vi "Result Response.vi"(8 "error in (no error)":errorcluster, 10 "Acquired Result.lvclass":refnum<class "Acquired Result.lvclass">, 11 "Monitor Controller in":refnum<class "Monitor Controller.lvclass">) -> (0 "error out":errorcluster, 3 "Monitor Controller out":refnum<class "Monitor Controller.lvclass">)   [LabVIEW 2016, in "Monitor Controller.lvclass"]
uses:
  Monitor Controller.lvclass
  D:/github/Measure_core/Da Base/Da Base.lvclass
  D:/Program Files/National Instruments/LabVIEW 2016/vi.lib/ActorFramework/Actor/Actor.lvclass
  Results/Acquired Result/Acquired Result.lvclass
  Monitor Controller.lvclass/Monitor Controller.ctl
  Da Base/Da Base.lvclass/Da Base.ctl
  <vilib>/ActorFramework/Actor/Actor.lvclass/Actor.ctl
  Process Controller Messages/Update Plots Msg/Update Plots Msg.lvclass/Update Plots Msg.ctl
  <vilib>/ActorFramework/Message Enqueuer/Message Enqueuer.lvclass/Message Enqueuer.ctl
  da Base/Read tdms stream.vi
  <vilib>/ActorFramework/Message Enqueuer/Enqueue.vi
  Process Controller Messages/Update Plots Msg/Update Plots Msg.lvclass
  D:/Program Files/National Instruments/LabVIEW 2016/vi.lib/ActorFramework/Message/Message.lvclass
  Read Monitor controller configuration.vi
  <vilib>/ActorFramework/Message Priority Queue/Priority Enqueue.vi
  Process Controller/Process Controller.lvclass
  <vilib>/ActorFramework/Actor/Actor.lvclass
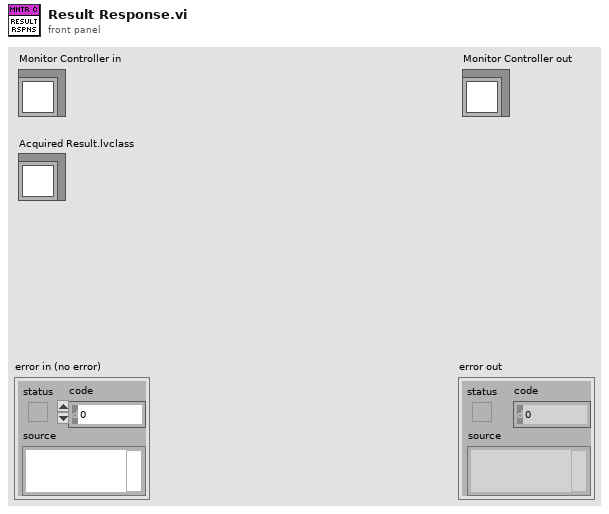
[diagram p1: front panel]
types:
  T1 = typedef "Monitor Controller Configuration.ctl" = cluster{"Period":dbl, "Repeat times":i32, "Open plot":bool, "File defragment period":dbl}
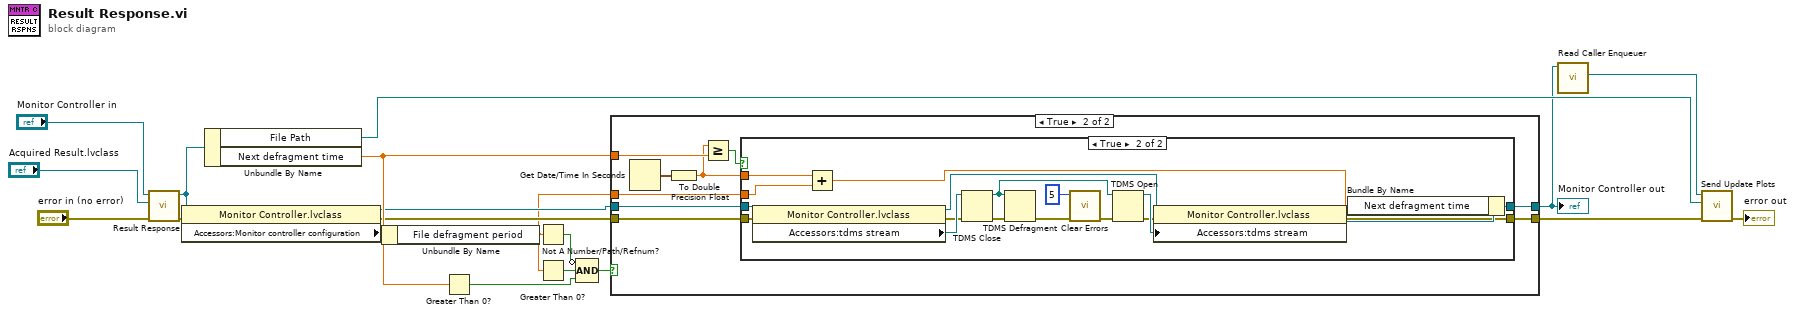
[diagram p0: block diagram]
diagram:
  n1 = call-parent "Result Response.vi"("error in (no error)"="error in (no error)", "Acquired Result"="Acquired Result.lvclass", "Measure Controller in"="Monitor Controller in") -> ("error out"=w2:errorcluster, "Measure Controller out"=w14:refnum<class "Monitor Controller.lvclass">)  [unwired: 7 in]
  n2 = property class="Monitor Controller.lvclass"(reference=w14, error in=w2) -> (reference out=w7:refnum<class "Monitor Controller.lvclass">, error out=w6:errorcluster, "Accessors:Monitor controller configuration"=w13:T1)
  n3 = Unbundle By Name(w14) -> ("File Path"=w15:path, "Next defragment time"=w8:dbl)
  n4 = Unbundle By Name(w13) -> ("File defragment period"=w5:dbl)
  n5 = Greater Than 0?(x=w8) -> (x > 0?=w9:bool)
  n6 = Not A Number/Path/Refnum?(number/path/refnum=w5) -> (NaN/Path/Refnum?=w11:bool)
  n7 = Greater Than 0?(x=w5) -> (x > 0?=w12:bool)
  n8 = Compound Arithmetic op=AND(invert w11, w12, w9) -> (w10:bool)
  n9 = case shown="True" w10 {
    tunnel: w8 -> [_ w29]
    tunnel: w7 -> [w21 w27]
    tunnel: w6 -> [w20 w26]
    tunnel: w5 -> [_ w24]
    tunnel: [w21 w23] -> w1
    tunnel: [w20 w22] -> w4
    frame False {
    }
    frame True {
      n10 = Get Date/Time In Seconds() -> (seconds since 1Jan1904=w30:timestamp)
      n11 = To Double Precision Float(number=w30) -> (double precision float=w25:dbl)
      n12 = Greater Or Equal?(x=w25, y=w29) -> (x >= y?=w28:bool)
      n13 = case shown="True" w28 {
        tunnel: w27 -> [w32 w50]
        tunnel: w26 -> [w31 w49]
        tunnel: w25 -> [_ w40]
        tunnel: w24 -> [_ w39]
        tunnel: [w32 w36] -> w23
        tunnel: [w31 w35] -> w22
        frame False {
        }
        frame True {
          n14 = property class="Monitor Controller.lvclass"(reference=w50, error in=w49) -> (reference out=w43:refnum<class "Monitor Controller.lvclass">, error out=w47:errorcluster, "Accessors:tdms stream"=w48:refnum<k34>)
          n15 = Add(x=w40, y=w39) -> (x+y=w37:dbl)
          n16 = TDMS Close(8:w47, 11:w48) -> (0:w46:errorcluster, 3:w44:path)
          n17 = TDMS Defragment(4:w46, 7:w44) -> (0:w45:errorcluster)
          n18 = call <vilib>:"Clear Errors.vi"("error in (no error)"=w45, "specific error code to clear (0: all)"=5) -> ("error out"=w34:errorcluster)  [unwired: 4 in, 1 out]
          n19 = TDMS Open(8:w34, 11:w44) -> (0:w41:errorcluster, 3:w42:refnum<k34>)  [unwired: 5 in]
          n20 = property class="Monitor Controller.lvclass"(reference=w43, error in=w41, "Accessors:tdms stream"=w42) -> (reference out=w38:refnum<class "Monitor Controller.lvclass">, error out=w35:errorcluster)
          n21 = Bundle By Name(cluster=w38, "Next defragment time"=w37) -> (w36:refnum<class "Monitor Controller.lvclass">)
        }
      }
    }
  }
  "Monitor Controller out" <- w1
  n22 = call <vilib>:"Read Caller Enqueuer.vi"("Actor"=w1) -> ("Caller Enqueuer"=w16:refnum<class "Message Enqueuer.lvclass">)  [unwired: 10 in]
  n23 = call "Send Update Plots.vi"("error in (no error)"=w4, "File Path"=w15, "Message Enqueuer"=w16) -> ("error out"=→"error out":errorcluster)  [unwired: 7 in, 1 out]
